vi "DFH.vi"(0 "System no.":i32=1 min=1 max=4 step=1, 2 "DFH axes":string[](array[string]), 3 "All axes?":bool, 4 "Axis identifier?":bool=TRUE, 5 "error in":errorcluster) -> (19 "error out":errorcluster)   [LabVIEW 2020]
doc: "Defines current position of the \"DFH axes\" as home position. Their position value is set to 0. Due to the change of the home position the values for the travel range limits (TMN?, TMX?) are also changed accordingly. The home position is reset to default by ATZ.vi, REF.vi, MNL.vi, MPL.vi or similiar command VIs.\n\nC-867, Mercury_GCS: If All axes? = TRUE, then Axis identifier? must be TRUE. \n\nC-880K005: VI only supported when called through PI_Multix.vi\n\nE-517: If All axes? = TRUE, then Axis identifier? must be TRUE. The values are saved with WPA 100. The position shown in the E-517 display is not affected by DFH because it is that of the sensor channel (can also be queried with TSP?). DFH affects only the axis position which can be queried with POS?.\n\nE-755: If All axes? = TRUE, then Axis identifier? must be TRUE. Command not available for E-755.101.\n\nE-518, E-761: If All axes? = TRUE, then Axis identifier? must be TRUE. The values are saved with WPA 100.\n\nAll other systems: If All axes? = TRUE, then Axis identifier? must be TRUE"
panel:
  # "Defines current position of the \"DFH axes\" as home \nposition. Their position value is set to 0. The home\nposition is reset to default by \"ATZ.vi\", \"REF.vi\", \n\"MNL.vi\", \"MPL.vi\" or similiar command VIs."
  # "If all axes: use"
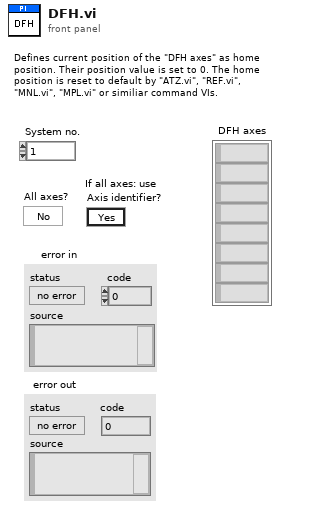
[diagram p1: front panel]
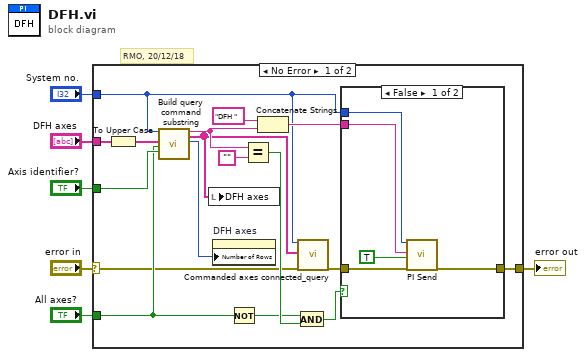
[diagram p0: block diagram]
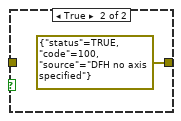
[diagram p2: hidden frame]
diagram:
  # "RMO, 20/12/18"
  n1 = case shown="No Error" "error in" {
    selector: "error in" -> [w7 w30]
    tunnel: "DFH axes" -> [w22 _]
    tunnel: "Axis identifier?" -> [w19 _]
    tunnel: "System no." -> [w8 _]
    tunnel: "All axes?" -> [w14 _]
    tunnel: [w11 w30] -> w2
    frame No Error {
      n2 = To Upper Case(1:w22) -> (0:w20:string[])
      n3 = call "Build query command substring.vi"("System no."=w8, "Axes to query in"=w20, "Query\nAll axes?"=w14, "For all axes: use\nAxis identifier?"=w19) -> ("Command substring"=w18:string, "Axes to query out"=w17:string[], "Number of rows"=w16:u32)  [unwired: 2 in, 11 out]
      n4 = local write "DFH axes"(w17) -> ()
      n5 = property on="DFH axes" class="Arr (strict)"("Number of Rows"=w16) -> ()  [unwired: 2 in, 2 out]
      n6 = Not(x=w14) -> (.not. x?=w13:bool)
      n7 = Equal?(x=w18, y="" ("x")) -> (x = y?=w15:bool)
      n8 = Concatenate Strings("DFH ", w18) -> (w9:string)
      n9 = And(x=w13, y=w15) -> (x .and. y?=w12:bool)
      n10 = call "Commanded axes connected_query.vi"("System no."=w8, "Commanded axes"=w17, "error in"=w7) -> ("error out"=w10:errorcluster)  [unwired: 1 in, 15 out]
      n11 = case shown="False" w12 {
        tunnel: [w27 errorcluster {"status"=TRUE, "code"=100, "source"="DFH no axis specified"} ("error out")] -> w11
        tunnel: w10 -> [w28 _]
        tunnel: w9 -> [w25 _]
        tunnel: w8 -> [w24 _]
        frame False {
          n12 = call "PI Send.vi"("System no."=w24, "String to send"=w25, "Attach termination char.?"=TRUE ("Attach Linefeed?"), "error in"=w28) -> ("error out"=w27:errorcluster)  [unwired: 2 in, 13 out]
        }
        frame True {
        }
      }
    }
    frame Error {
    }
  }
  "error out" <- w2
